vi "保持寄存器解析.vi"(11 "A读保持寄存器信息组":T2(array[cluster])=[{"地址"=10099, "数量"=2, "寄存器值"=[0, 0], "名称"="产品总数"}, {"地址"=10101, "数量"=2, "寄存器值"=[0, 0], "名称"="合格数量"}, {"地址"=10103, "数量"=2, "寄存器值"=[0, 0], "名称"="泄露数量"}, {"地址"=506, "数量"=2, "寄存器值"=[0, 0], "名称"="1测试时间"}, {"地址"=508, "数量"=2, "寄存器值"=[0, 0], "名称"="1测试泄漏"}, {"地址"=1506, "数量"=2, "寄存器值"=[0, 0], "名称"="2测试时间"}, {"地址"=1508, "数量"=2, "寄存器值"=[0, 0], "名称"="2采样泄漏"}, {"地址"=504, "数量"=2, "寄存器值"=[0, 0], "名称"="1#目标压力"}, {"地址"=498, "数量"=1, "寄存器值"=[0, 0], "名称"="1#测试结果"}, {"地址"=1498, "数量"=1, "寄存器值"=[0, 64], "名称"="2#测试结果"}, {"地址"=1504, "数量"=2, "寄存器值"=[0, 0], "名称"="2#目标压力"}, {"地址"=500, "数量"=1, "寄存器值"=[0], "名称"="实时压力"}] {"寄存器值" format="%x"}) -> (2 "运行状态":string, 3 "参数值":T1(array[cluster]))   [LabVIEW 2020]
panel:
  out "泄漏流量":dbl
  out "参数组别":u32
  out "测试时间":dbl
  out "参数值":string[](array[string])
  out "失败原因":string
  out "1OK":bool
  out "测试结果  1":string
  out "门限压力":i32
  out "实时压力":i32
  out "目标压力":i32
  out "泄漏压力":dbl
  out "NG":u32
  out "OK":u32
  out "总量":u32
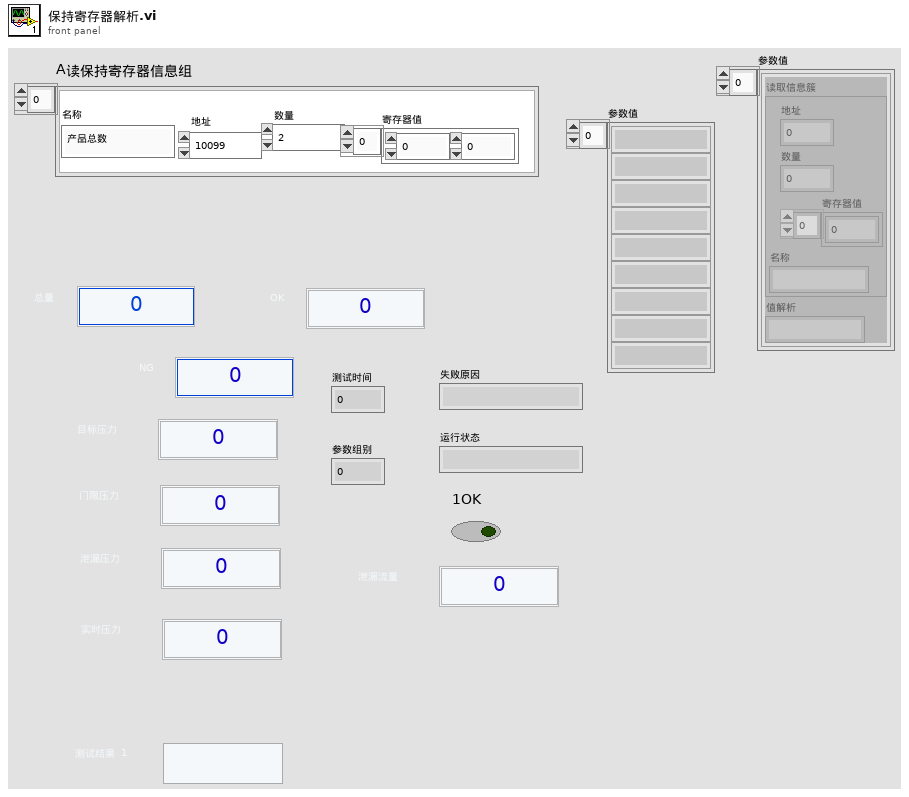
[diagram p1: front panel]
types:
  T1 = cluster{"读取信息簇":cluster{"地址":u16, "数量":u16, "寄存器值":u16[], "名称":string}, "值解析":string}[]
  T2 = cluster{"地址":u16, "数量":u16, "寄存器值":u16[], "名称":string}[]
  T3 = cluster{"读取信息簇":cluster{"地址":u16, "数量":u16, "寄存器值":u16[], "名称":string}, "值解析":string}
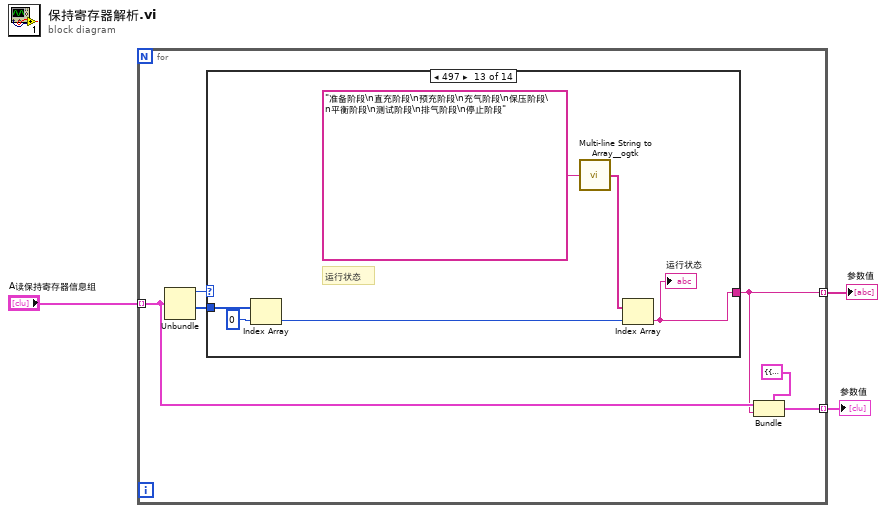
[diagram p0: block diagram]
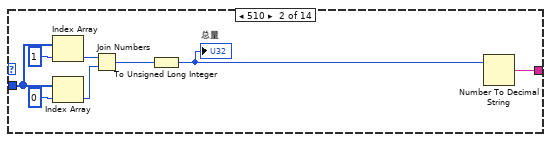
[diagram p3: hidden frame]
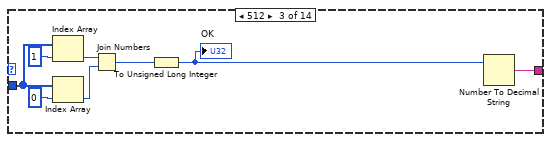
[diagram p4: hidden frame]
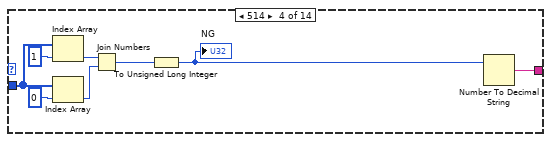
[diagram p5: hidden frame]
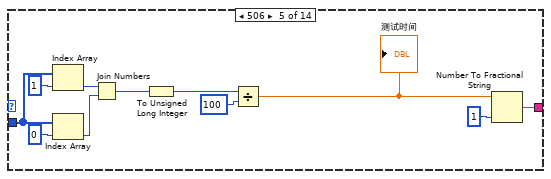
[diagram p6: hidden frame]
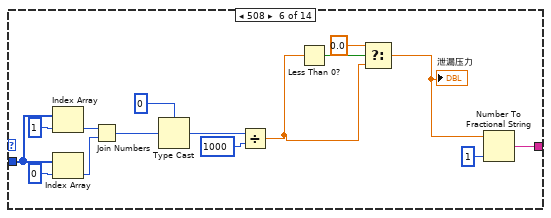
[diagram p7: hidden frame]
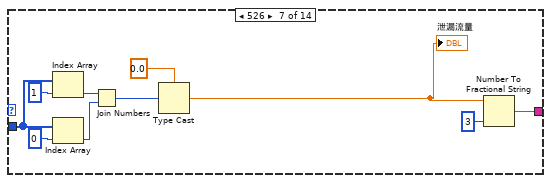
[diagram p8: hidden frame]
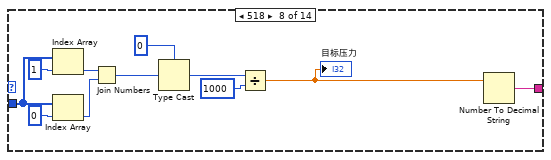
[diagram p9: hidden frame]
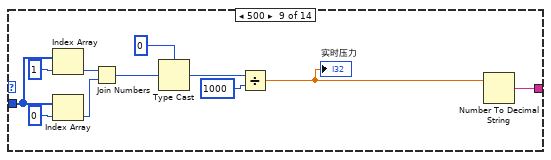
[diagram p10: hidden frame]
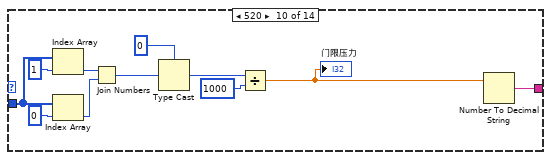
[diagram p11: hidden frame]
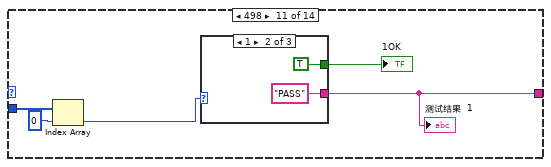
[diagram p12: hidden frame]
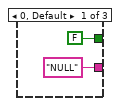
[diagram p13: hidden frame]
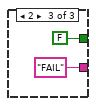
[diagram p14: hidden frame]
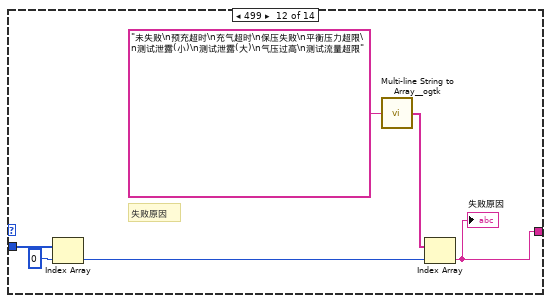
[diagram p15: hidden frame]
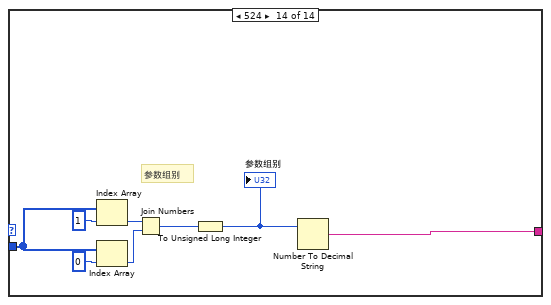
[diagram p16: hidden frame]
diagram:
  n1 = for {
    tunnel: "A读保持寄存器信息组" -> [w7] mode=indexing
    tunnel: [w6] -> w2 mode=indexing
    tunnel: [w5] -> w1 mode=indexing
    n2 = Unbundle(w7) -> ("地址"=w9:u16, "寄存器值"=w8:u16[])  [unwired: 2 out]
    n3 = case shown="497" w9 {
      tunnel: w8 -> [_ w16 w24 w32 w43 w58 w68 w74 w85 w96 w106 w118 w124 w128]
      tunnel: [_ w10 w18 w26 w34 w50 w62 w70 w81 w92 w103 w114 w120 w127] -> w6
      frame Default {
      }
      frame 510 {
        n4 = Index Array(array=w16, index=1 ("索引")) -> (element=w14:u16)
        n5 = Index Array(array=w16, index=0 ("索引")) -> (element=w13:u16)
        n6 = Join Numbers(hi=w14, lo=w13) -> ((hi.lo)=w12:u32)
        n7 = To Unsigned Long Integer(number=w12) -> (unsigned 32bit integer=w11:u32)
        "总量" <- w11
        n8 = Number To Decimal String(number=w11) -> (decimal integer string=w10:string)  [unwired: 1 in]
      }
      frame 512 {
        n9 = Index Array(array=w24, index=1 ("索引")) -> (element=w22:u16)
        n10 = Index Array(array=w24, index=0 ("索引")) -> (element=w21:u16)
        n11 = Join Numbers(hi=w22, lo=w21) -> ((hi.lo)=w20:u32)
        n12 = To Unsigned Long Integer(number=w20) -> (unsigned 32bit integer=w19:u32)
        "OK" <- w19
        n13 = Number To Decimal String(number=w19) -> (decimal integer string=w18:string)  [unwired: 1 in]
      }
      frame 514 {
        n14 = Index Array(array=w32, index=1 ("索引")) -> (element=w30:u16)
        n15 = Index Array(array=w32, index=0 ("索引")) -> (element=w29:u16)
        n16 = Join Numbers(hi=w30, lo=w29) -> ((hi.lo)=w28:u32)
        n17 = To Unsigned Long Integer(number=w28) -> (unsigned 32bit integer=w27:u32)
        "NG" <- w27
        n18 = Number To Decimal String(number=w27) -> (decimal integer string=w26:string)  [unwired: 1 in]
      }
      frame 506 {
        n19 = Index Array(array=w43, index=1 ("索引")) -> (element=w41:u16)
        n20 = Index Array(array=w43, index=0 ("索引")) -> (element=w40:u16)
        n21 = Join Numbers(hi=w41, lo=w40) -> ((hi.lo)=w39:u32)
        n22 = To Unsigned Long Integer(number=w39) -> (unsigned 32bit integer=w38:u32)
        n23 = Divide(x=w38, y=u32 100) -> (x/y=w36:dbl)
        "测试时间" <- w36
        n24 = Number To Fractional String(number=w36, precision (6)=i16 1 ("精度(6)")) -> (F-format string=w34:string)  [unwired: 2 in]
      }
      frame 508 {
        n25 = Index Array(array=w58, index=1 ("索引")) -> (element=w56:u16)
        n26 = Index Array(array=w58, index=0 ("索引")) -> (element=w55:u16)
        n27 = Join Numbers(hi=w56, lo=w55) -> ((hi.lo)=w54:u32)
        n28 = Type Cast(type=0 ("泄漏压力"), x=w54) -> (*(type *) &x=w51:i32)
        n29 = Divide(x=w51, y=u32 1000) -> (x/y=w46:dbl)
        n30 = Less Than 0?(x=w46) -> (x < 0?=w48:bool)
        n31 = Select(t=0.0, s=w48, f=w46) -> (s? t:f=w45:dbl)
        "泄漏压力" <- w45
        n32 = Number To Fractional String(number=w45, precision (6)=i16 1 ("精度(6)")) -> (F-format string=w50:string)  [unwired: 2 in]
      }
      frame 526 {
        n33 = Index Array(array=w68, index=1 ("索引")) -> (element=w66:u16)
        n34 = Index Array(array=w68, index=0 ("索引")) -> (element=w65:u16)
        n35 = Join Numbers(hi=w66, lo=w65) -> ((hi.lo)=w64:u32)
        n36 = Type Cast(type=sgl 0.0 ("泄漏压力"), x=w64) -> (*(type *) &x=w60:sgl)
        "泄漏流量" <- w60
        n37 = Number To Fractional String(number=w60, precision (6)=i16 3 ("精度(6)")) -> (F-format string=w62:string)  [unwired: 2 in]
      }
      frame 518 {
        n38 = Index Array(array=w74, index=1 ("索引")) -> (element=w80:u16)
        n39 = Index Array(array=w74, index=0 ("索引")) -> (element=w79:u16)
        n40 = Join Numbers(hi=w80, lo=w79) -> ((hi.lo)=w78:u32)
        n41 = Type Cast(type=0 ("泄漏压力"), x=w78) -> (*(type *) &x=w72:i32)
        n42 = Divide(x=w72, y=u32 1000) -> (x/y=w71:dbl)
        "目标压力" <- w71
        n43 = Number To Decimal String(number=w71) -> (decimal integer string=w70:string)  [unwired: 1 in]
      }
      frame 500 {
        n44 = Index Array(array=w85, index=1 ("索引")) -> (element=w91:u16)
        n45 = Index Array(array=w85, index=0 ("索引")) -> (element=w90:u16)
        n46 = Join Numbers(hi=w91, lo=w90) -> ((hi.lo)=w89:u32)
        n47 = Type Cast(type=0 ("泄漏压力"), x=w89) -> (*(type *) &x=w83:i32)
        n48 = Divide(x=w83, y=u32 1000) -> (x/y=w82:dbl)
        "实时压力" <- w82
        n49 = Number To Decimal String(number=w82) -> (decimal integer string=w81:string)  [unwired: 1 in]
      }
      frame 520 {
        n50 = Index Array(array=w96, index=1 ("索引")) -> (element=w102:u16)
        n51 = Index Array(array=w96, index=0 ("索引")) -> (element=w101:u16)
        n52 = Join Numbers(hi=w102, lo=w101) -> ((hi.lo)=w100:u32)
        n53 = Type Cast(type=0 ("泄漏压力"), x=w100) -> (*(type *) &x=w94:i32)
        n54 = Divide(x=w94, y=u32 1000) -> (x/y=w93:dbl)
        "门限压力" <- w93
        n55 = Number To Decimal String(number=w93) -> (decimal integer string=w92:string)  [unwired: 1 in]
      }
      frame 498 {
        n56 = Index Array(array=w106, index=0 ("索引")) -> (element=w104:u16)
        n57 = case shown="1" w104 {
          tunnel: [FALSE ("1OK") TRUE ("1OK") FALSE ("1OK")] -> w105
          tunnel: ["NULL" ("格式字符串") "PASS" ("格式字符串") "FAIL" ("格式字符串")] -> w103
          frame 0, Default {
          }
          frame 1 {
          }
          frame 2 {
          }
        }
        "1OK" <- w105
        "测试结果  1" <- w103
      }
      frame 499 {
        # "失败原因"
        n58 = Index Array(array=w118, index=0 ("索引")) -> (element=w115:u16)
        n59 = call <userlib>:"Multi-line String to Array__ogtk.vi"("string"="未失败\n预充超时\n充气超时\n保压失败\n平衡压力超限\n测试泄露(小)\n测试泄露(大)\n气压过高\n测试流量超限") -> ("lines"=w116:string[])
        n60 = Index Array(array=w116, index=w115) -> (element=w114:string)
        "失败原因" <- w114
      }
      frame 497 {
        # "运行状态"
        n61 = Index Array(array=w124, index=0 ("索引")) -> (element=w121:u16)
        n62 = call <userlib>:"Multi-line String to Array__ogtk.vi"("string"="准备阶段\n直充阶段\n预充阶段\n充气阶段\n保压阶段\n平衡阶段\n测试阶段\n排气阶段\n停止阶段") -> ("lines"=w122:string[])
        n63 = Index Array(array=w122, index=w121) -> (element=w120:string)
        "运行状态" <- w120
      }
      frame 524 {
        # "参数组别"
        n64 = Index Array(array=w128, index=1 ("索引")) -> (element=w131:u16)
        n65 = Index Array(array=w128, index=0 ("索引")) -> (element=w130:u16)
        n66 = Join Numbers(hi=w131, lo=w130) -> ((hi.lo)=w129:u32)
        n67 = To Unsigned Long Integer(number=w129) -> (unsigned 32bit integer=w126:u32)
        "参数组别" <- w126
        n68 = Number To Decimal String(number=w126) -> (decimal integer string=w127:string)  [unwired: 1 in]
      }
    }
    n69 = Bundle(cluster=T3 {"读取信息簇"={"地址"=0, "数量"=0, "寄存器值"=[], "名称"=""}, "值解析"=""} ("簇"), "读取信息簇"=w7, "值解析"=w6) -> (w5:T3)
  }
  "参数值" <- w2
  "参数值" <- w1
